vi "Read Wash Display Console.vi"(8 "error in (no error)":errorcluster, 11 "Simulation Interface in":refnum<class "Simulation Interface.lvclass">) -> (0 "error out":errorcluster, 2 "Wash Display Console.lvlib:Wash Display Console.lvclass":refnum<class "Wash Display Console.lvclass">, 3 "Simulation Interface out":refnum<class "Simulation Interface.lvclass">)   [LabVIEW 2012, in "Simulation Interface.lvclass"]
uses:
  Simulation Interface.lvclass
  Wash Display Console/Wash Display Console.lvclass
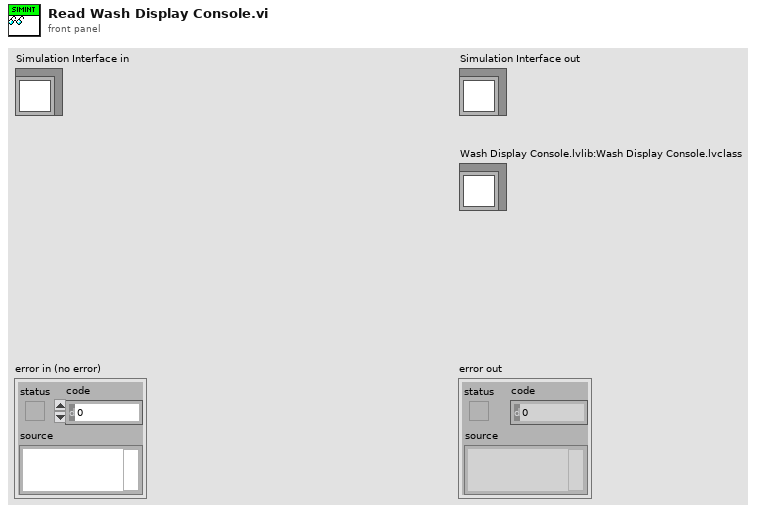
[diagram p1: front panel]
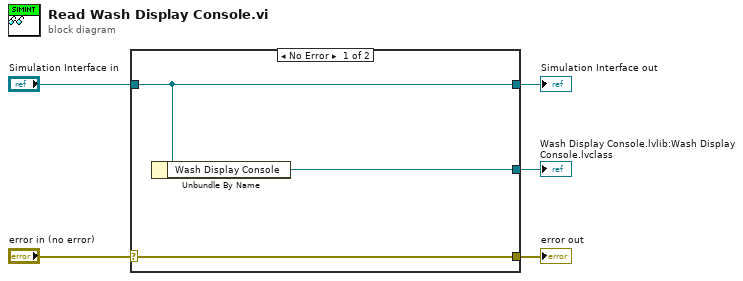
[diagram p0: block diagram]
diagram:
  n1 = case shown="No Error" "error in (no error)" {
    selector: "error in (no error)" -> [w8 w9]
    tunnel: [w8 w9] -> w4
    tunnel: [w7 w10] -> w2
    tunnel: "Simulation Interface in" -> [w7 w10]
    tunnel: [w6 _] -> w1
    frame No Error {
      n2 = Unbundle By Name(w7) -> ("Wash Display Console"=w6:refnum<class "Wash Display Console.lvclass">)
    }
    frame Error {
    }
  }
  "error out" <- w4
  "Simulation Interface out" <- w2
  "Wash Display Console.lvlib:Wash Display Console.lvclass" <- w1
